vi "test9-LocalExternalStateRegistrationViaAPI.vi"(8 "error in (no error)":errorcluster, 11 "TestCase in":refnum<class "testcase-CSMBroadcast.lvclass">) -> (0 "error out":errorcluster, 3 "TestCase out":refnum<class "testcase-CSMBroadcast.lvclass">)   [LabVIEW 2017, in "testcase-CSMBroadcast.lvclass"]
uses:
  testcase-CSMBroadcast.lvclass
  0b17d103-e67b-41be-a9eb-a2ee1311ff1f.vi
  5999693e-4f8a-4b34-ae87-f34dff5771be.vi
  52a2a10a-a04b-4bad-8df4-e1eb944f47cc.vi
  826f03dd-b4b5-4c6b-9085-8edf6da4f43b.vi
  src/user.lib/_NEVSTOP/Communicable State Machine(CSM)/AdvanceAPI/CSM - Get Module Attribute.vi
  <vilib>/addons/_JKI Toolkits/VI Tester/TestCase.llb/TestCase.lvclass
  src/user.lib/_NEVSTOP/Communicable State Machine(CSM)/Communicable State Machine.lvlib
  C:/Program Files (x86)/National Instruments/LabVIEW 2017/vi.lib/addons/_JKI Toolkits/VI Tester/TestCase.llb/TestCase.lvclass
panel:
  out "LoopCount 2":i32
  out "LoopCount":i32
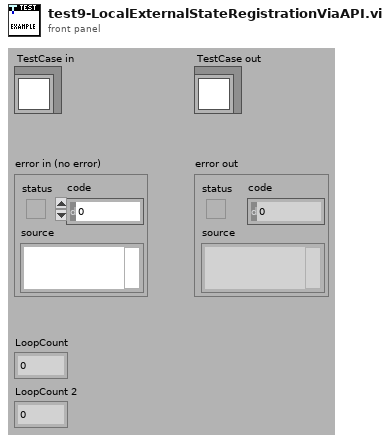
[diagram p1: front panel]
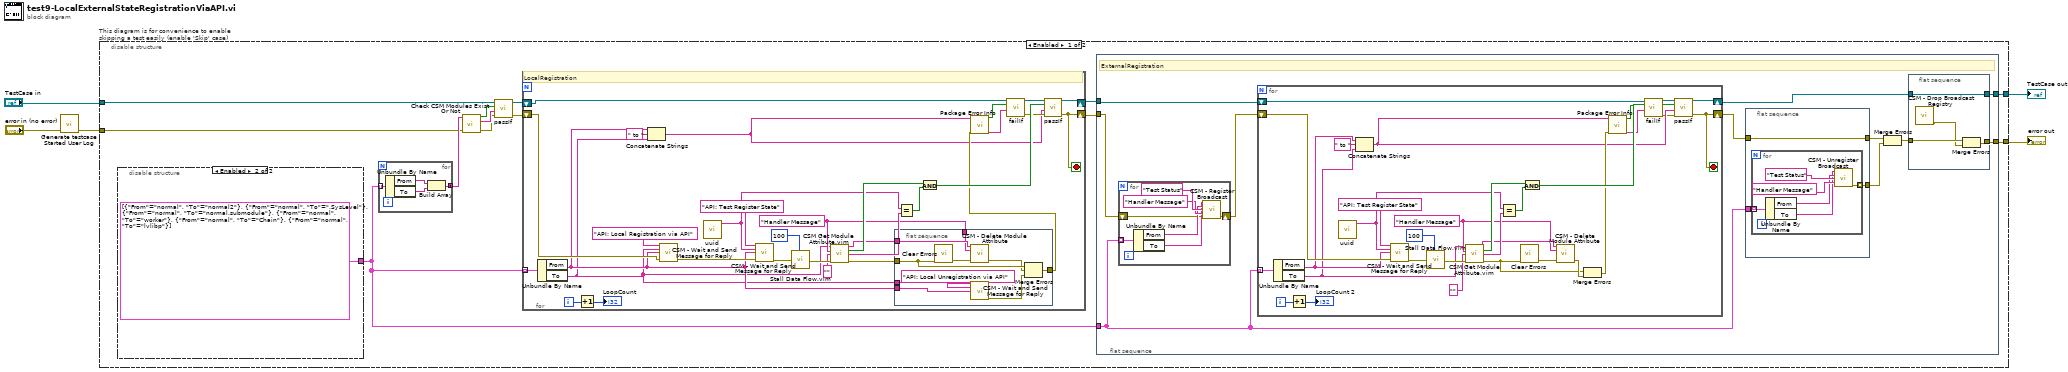
[diagram p0: block diagram]
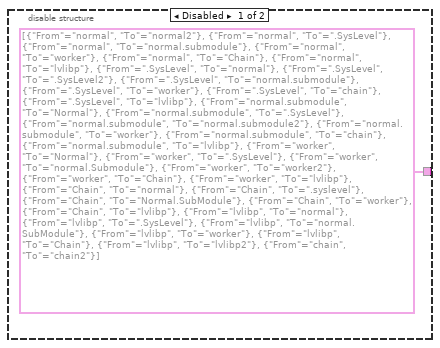
[diagram p2: hidden frame]
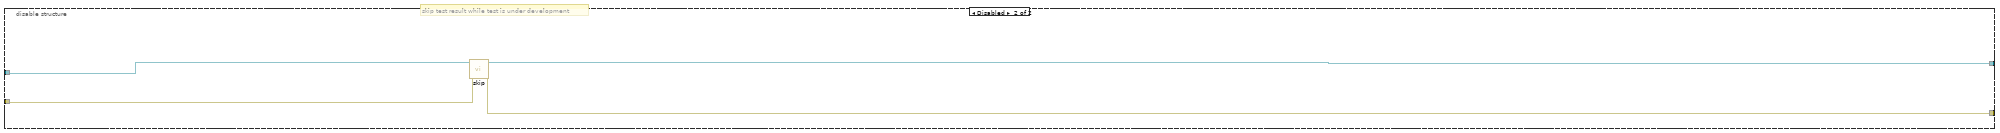
[diagram p3: hidden frame]
diagram:
  n1 = call "Generate testcase Started User Log.vi"("Error In"="error in (no error)") -> ("error out"=w1:errorcluster)  [unwired: 10 in]
  n2 = disable-structure "This diagram is for convenience to enable skipping a test easily (enable 'Skip' case)" shown="Enabled" {
    disable-tunnel: "TestCase in" -> [w8 w131]
    disable-tunnel: [w17 w129] -> w2
    disable-tunnel: [w15 w130] -> w4
    disable-tunnel: w1 -> [w7 w128]
    frame Enabled {
      n3 = disable-structure shown="Enabled" {
        disable-tunnel: [cluster{"From":string, "To":string}[] [{"From"="normal", "To"="normal2"}, {"From"="normal", "To"=".SysLevel"}, {"From"="normal", "To"="normal.submodule"}, {"From"="normal", "To"="worker"}, {"From"="normal", "To"="Chain"}, {"From"="normal", "To"="lvlibp"}, {"From"=".SysLevel", "To"="normal"}, {"From"=".SysLevel", "To"=".SysLevel2"}, {"From"=".SysLevel", "To"="normal.submodule"}, {"From"=".SysLevel", "To"="worker"}, {"From"=".SysLevel", "To"="chain"}, {"From"=".SysLevel", "To"="lvlibp"}, {"From"="normal.submodule", "To"="Normal"}, {"From"="normal.submodule", "To"=".SysLevel"}, {"From"="normal.submodule", "To"="normal.submodule2"}, {"From"="normal.submodule", "To"="worker"}, {"From"="normal.submodule", "To"="chain"}, {"From"="normal.submodule", "To"="lvlibp"}, {"From"="worker", "To"="Normal"}, {"From"="worker", "To"=".SysLevel"}, {"From"="worker", "To"="normal.Submodule"}, {"From"="worker", "To"="worker2"}, {"From"="worker", "To"="Chain"}, {"From"="worker", "To"="lvlibp"}, {"From"="Chain", "To"="normal"}, {"From"="Chain", "To"=".syslevel"}, {"From"="Chain", "To"="Normal.SubModule"}, {"From"="Chain", "To"="worker"}, {"From"="Chain", "To"="lvlibp"}, {"From"="lvlibp", "To"="normal"}, {"From"="lvlibp", "To"=".SysLevel"}, {"From"="lvlibp", "To"="normal.SubModule"}, {"From"="lvlibp", "To"="worker"}, {"From"="lvlibp", "To"="Chain"}, {"From"="lvlibp", "To"="lvlibp2"}, {"From"="chain", "To"="chain2"}] cluster{"From":string, "To":string}[] [{"From"="normal", "To"="normal2"}, {"From"="normal", "To"=".SysLevel"}, {"From"="normal", "To"="normal.submodule"}, {"From"="normal", "To"="worker"}, {"From"="normal", "To"="Chain"}, {"From"="normal", "To"="lvlibp"}]] -> w6
        frame Disabled {
        }
        frame Enabled {
        }
      }
      n4 = for {
        tunnel: w6 -> [w24] mode=indexing
        tunnel: [w21] -> w13 mode=concatenating
        n5 = Unbundle By Name(w24) -> ("From"=w23:string, "To"=w22:string)
        n6 = Build Array(w23, w22) -> (w21:string[])
      }
      n7 = call "Check CSM Modules Exist Or Not.vi"("error in"=w7, "CSM names in"=w13) -> ("error out"=w11:errorcluster, "Debug string"=w12:string, "All Modules Exist?"=w14:bool)  [unwired: 7 in]
      n8 = call-dynamic "passIf.vi"("error in (no error)"=w11, "message (\"\")"=w12, "pass"=w14, "TestCase in"=w8) -> ("error out"=w10:errorcluster, "TestCase out"=w9:refnum<class "testcase-CSMBroadcast.lvclass">)  [unwired: 6 in]
      n9 = for {
        shift-right: [w35] -> w16
        shift-left: w10 -> [w36]
        shift-right: [w42] -> w18
        shift-left: w9 -> [w32]
        tunnel: w6 -> [w53] mode=indexing
        i -> [w55]
        stop <- w35 stop-if-true
        w37 = "Handler Message" ("To")
        # "LocalRegistration"
        n10 = Unbundle By Name(w53) -> ("From"=w28:string, "To"=w27:string)
        n11 = Increment(x=w55) -> (x+1=→"LoopCount":i32)
        n12 = Concatenate Strings(w28, " to " ("string"), w27) -> (w25:string)
        n13 = call "CSM - Wait and Send Message for Reply.vi"("State"="API: Local Registration via API", "Arguments (\"\")"=w27, "Target Module"=w28, "Error In (No Error)"=w36) -> ("error out"=w50:errorcluster)  [unwired: 8 in, 3 out]
        n14 = call "uuid.vi"() -> ("UUID"=w44:string)  [unwired: 11 in]
        n15 = call "CSM - Wait and Send Message for Reply.vi"("State"="API: Test Register State", "Arguments (\"\")"=w44, "Target Module"=w28, "Error In (No Error)"=w50) -> ("error out"=w49:errorcluster)  [unwired: 8 in, 3 out]
        n16 = call "Stall Data Flow.vim"("value in"=w49, "milliseconds to wait"=u32 100) -> ("value out"=w47:errorcluster)  [unwired: 1 out]
        n17 = call "CSM Get Module Attribute.vim"("CSM Name"=w27, "Attribute"=w37, "Default Value (Empty Variant)"="", "Error In"=w47) -> ("CSM Name (Dup)"=w38:string, "Found"=w46:bool, "Value"=w43:string, "error out"=w39:errorcluster)  [unwired: 7 in, 1 out]
        n18 = flat-sequence {
          tunnel: w39 -> [w59]
          tunnel: w38 -> [w64]
          tunnel: w37 -> [w63]
          tunnel: w27 -> [w61]
          tunnel: w28 -> [w60]
          tunnel: [w56] -> w29
          frame #0 {
            n19 = call <vilib>:"Clear Errors.vi"("error in (no error)"=w59) -> ("error out"=w65:errorcluster)  [unwired: 5 in, 1 out]
            n20 = call "CSM - Delete Module Attribute.vi"("CSM Name"=w64, "Attribute"=w63, "Error In"=w65) -> ("error out"=w58:errorcluster)  [unwired: 9 in, 3 out]
            n21 = call "CSM - Wait and Send Message for Reply.vi"("State"="API: Local Unregistration via API", "Arguments (\"\")"=w61, "Target Module"=w60) -> ("error out"=w57:errorcluster)  [unwired: 9 in, 3 out]
            n22 = Merge Errors(w59, w58, w57) -> (w56:errorcluster)
          }
        }
        n23 = Equal?(x=w44, y=w43) -> (x = y?=w41:bool)
        n24 = And(x=w46, y=w41) -> (x .and. y?=w40:bool)
        n25 = call "Package Error Info.vi"("error in"=w29, "String in"=w25) -> ("packed error info out"=w33:string, "error status"=w34:bool)  [unwired: 8 in]
        n26 = call-dynamic "failIf.vi"("message (\"\")"=w33, "fail"=w34, "TestCase in"=w32) -> ("error out"=w30:errorcluster, "TestCase out"=w31:refnum<class "testcase-CSMBroadcast.lvclass">)  [unwired: 7 in]
        n27 = call-dynamic "passIf.vi"("error in (no error)"=w30, "message (\"\")"=w25, "pass"=w40, "TestCase in"=w31) -> ("error out"=w35:errorcluster, "TestCase out"=w42:refnum<class "testcase-CSMBroadcast.lvclass">)  [unwired: 6 in]
      }
      n28 = flat-sequence {
        tunnel: w18 -> [w76]
        tunnel: [w70] -> w17
        tunnel: w16 -> [w67]
        tunnel: w6 -> [w75]
        tunnel: [w72] -> w15
        frame #0 {
          # "ExternalRegistration"
          n29 = for {
            tunnel: w75 -> [w96] mode=indexing
            shift-right: [w91] -> w66
            shift-left: w67 -> [w90]
            n30 = Unbundle By Name(w96) -> ("From"=w93:string, "To"=w92:string)
            n31 = call "CSM - Register Broadcast.vi"("CSM Name(Empty for Broadcast Event)"=w92, "Source CSM Name (* as Default)"=w93, "Trigger"="Test Status" ("Status"), "API (If \"\", Same as Trigger)"="Handler Message" ("Response Message (If \"\", Same as Source Message)"), "Error In"=w90) -> ("error out"=w91:errorcluster)  [unwired: 9 in, 1 out]
          }
          n32 = for {
            shift-right: [w110] -> w69
            shift-left: w66 -> [w109]
            shift-right: [w116] -> w71
            shift-left: w76 -> [w99]
            tunnel: w75 -> [w125] mode=indexing
            i -> [w127]
            stop <- w110 stop-if-true
            w111 = "Handler Message" ("To")
            n33 = Unbundle By Name(w125) -> ("From"=w102:string, "To"=w101:string)
            n34 = Increment(x=w127) -> (x+1=→"LoopCount 2":i32)
            n35 = call "uuid.vi"() -> ("UUID"=w118:string)  [unwired: 11 in]
            n36 = Concatenate Strings(w102, " to " ("string"), w101) -> (w100:string)
            n37 = call "CSM - Wait and Send Message for Reply.vi"("State"="API: Test Register State", "Arguments (\"\")"=w118, "Target Module"=w102, "Error In (No Error)"=w109) -> ("error out"=w123:errorcluster)  [unwired: 8 in, 3 out]
            n38 = call "Stall Data Flow.vim"("value in"=w123, "milliseconds to wait"=u32 100) -> ("value out"=w121:errorcluster)  [unwired: 1 out]
            n39 = call "CSM Get Module Attribute.vim"("CSM Name"=w101, "Attribute"=w111, "Default Value (Empty Variant)"="", "Error In"=w121) -> ("CSM Name (Dup)"=w112:string, "Found"=w120:bool, "Value"=w117:string, "error out"=w107:errorcluster)  [unwired: 7 in, 1 out]
            n40 = Equal?(x=w118, y=w117) -> (x = y?=w115:bool)
            n41 = call <vilib>:"Clear Errors.vi"("error in (no error)"=w107) -> ("error out"=w113:errorcluster)  [unwired: 5 in, 1 out]
            n42 = And(x=w120, y=w115) -> (x .and. y?=w114:bool)
            n43 = call "CSM - Delete Module Attribute.vi"("CSM Name"=w112, "Attribute"=w111, "Error In"=w113) -> ("error out"=w108:errorcluster)  [unwired: 9 in, 3 out]
            n44 = Merge Errors(w107, w108) -> (w104:errorcluster)
            n45 = call "Package Error Info.vi"("error in"=w104, "String in"=w100) -> ("packed error info out"=w105:string, "error status"=w106:bool)  [unwired: 8 in]
            n46 = call-dynamic "failIf.vi"("message (\"\")"=w105, "fail"=w106, "TestCase in"=w99) -> ("error out"=w97:errorcluster, "TestCase out"=w98:refnum<class "testcase-CSMBroadcast.lvclass">)  [unwired: 7 in]
            n47 = call-dynamic "passIf.vi"("error in (no error)"=w97, "message (\"\")"=w100, "pass"=w114, "TestCase in"=w98) -> ("error out"=w110:errorcluster, "TestCase out"=w116:refnum<class "testcase-CSMBroadcast.lvclass">)  [unwired: 6 in]
          }
          n48 = flat-sequence {
            tunnel: w75 -> [w79]
            tunnel: [w78] -> w74
            tunnel: w69 -> [w77]
            tunnel: [w77] -> w68
            frame #0 {
              n49 = for {
                tunnel: w79 -> [w85] mode=indexing
                tunnel: [w80] -> w78 mode=indexing
                n50 = Unbundle By Name(w85) -> ("From"=w82:string, "To"=w81:string)
                n51 = call "CSM - Unregister Broadcast.vi"("CSM Name(Empty for Broadcast Event)"=w81, "Source CSM Name (* as Default)"=w82, "Trigger"="Test Status" ("Status"), "API (\"*\" as Default)"="Handler Message" ("Response Message (If \"\", Same as Source Message)")) -> ("error out"=w80:errorcluster)  [unwired: 10 in, 1 out]
              }
            }
          }
          n52 = Merge Errors(w68, w74) -> (w73:errorcluster)
          n53 = flat-sequence {
            tunnel: w73 -> [w89]
            tunnel: [w88] -> w72
            tunnel: [w87] -> w70
            tunnel: w71 -> [w87]
            frame #0 {
              n54 = call "CSM - Drop Broadcast Registry.vi"() -> ("error out"=w86:errorcluster)  [unwired: 15 in]
              n55 = Merge Errors(w89, w86) -> (w88:errorcluster)
            }
          }
        }
      }
    }
    frame Disabled {
      # "skip test result while test is under development"
      n56 = call <vilib>:"skip.vi"("error in (no error)"=w128, "TestCase in"=w131) -> ("error out"=w130:errorcluster, "TestCase out"=w129:refnum<class "testcase-CSMBroadcast.lvclass">)  [unwired: 8 in]
    }
  }
  "error out" <- w4
  "TestCase out" <- w2
